vi "Laser349_RS232_Read_Status.vi"(8 "error in (no error)":errorcluster, 10 "Command Status":T1, 11 "Laser349 in":refnum<class "Laser349.lvclass">) -> (0 "error out":errorcluster, 2 "Result String":string, 3 "Laser349 out":refnum<class "Laser349.lvclass">)   [LabVIEW 2018, in "Laser349.lvclass"]
uses:
  Laser349.lvclass
  Ctl/_ctl_LaserCmd.ctl
  Laser349.lvclass/Laser349.ctl
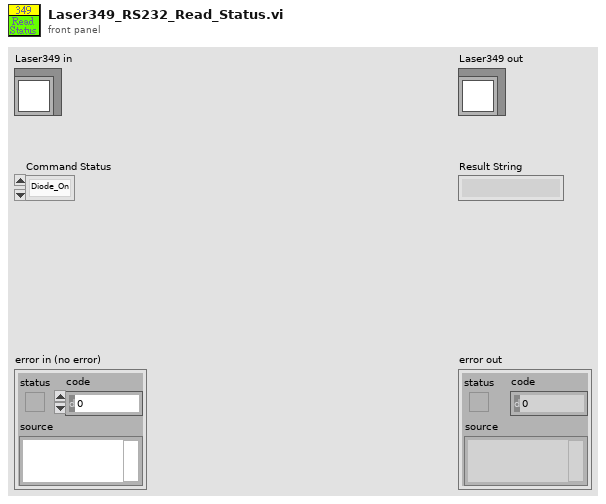
[diagram p1: front panel]
types:
  T1 = typedef "_ctl_LaserCmd.ctl" = enum8{"Diode_On", "Diode_Off", "Standby_On", "Standby_Off", "Internal_Trig", "External_Trig", "Set_Energy", "Set_Frequency", "Read_Version", "Read_STB", "Read_Diode_TEMP", "Read_SHG_TEMP", "Read_THG_TEMP", "Read_Base_Plate_TEMP", "Read_Diode_Hour", "Read_Diode_Maxc", "Read_Diode_Curr", "Read_QSW_CNTS", "Read_PENER", "Read_Freq", "Read_PCUR", "Read_Fault_Codes"}
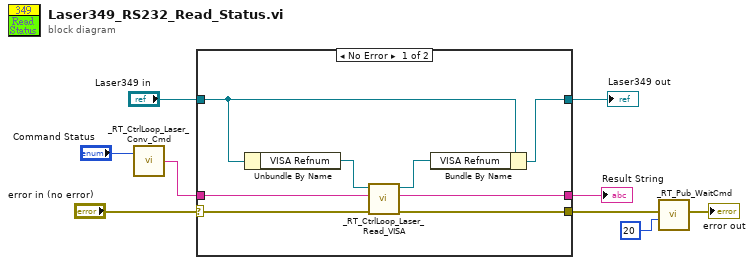
[diagram p0: block diagram]
diagram:
  n1 = call "_RT_CtrlLoop_Laser_Conv_Cmd.vi"("Command Status"="Command Status") -> ("Laser Command"=w1:string)  [unwired: 1 in]
  n2 = case shown="No Error" "error in (no error)" {
    selector: "error in (no error)" -> [w14 w19]
    tunnel: [w10 w19] -> w7
    tunnel: [w16 w18] -> w4
    tunnel: "Laser349 in" -> [w17 w18]
    tunnel: [w13 _] -> w3
    tunnel: w1 -> [w15 _]
    frame No Error {
      n3 = Unbundle By Name(w17) -> ("VISA Refnum"=w12:refnum<visa-resource-name>)
      n4 = call "_RT_CtrlLoop_Laser_Read_VISA.vi"("error in (no error)"=w14, "Comm Str"=w15, "VISA resource In"=w12) -> ("error out"=w10:errorcluster, "Response Str"=w13:string, "VISA resource Out"=w11:refnum<visa-resource-name>)  [unwired: 6 in]
      n5 = Bundle By Name(cluster=w17, "VISA Refnum"=w11) -> (w16:refnum<class "Laser349.lvclass">)
    }
    frame Error {
    }
  }
  "Laser349 out" <- w4
  "Result String" <- w3
  n6 = call "_RT_Pub_WaitCmd.vi"("milliseconds to wait"=u32 20, "error in (no error)"=w7) -> ("error out"=→"error out":errorcluster)  [unwired: 9 in]
